vi "Write Configuration to File.vi"(8 "error in":errorcluster, 11 "?":T1={"Data Tree Ref"=refnum, "FP Ref"=refnum, "Column Data Type"=[], "Search Clones Up To"=0, "SortOptions"={"Col.pri"=0, "RevDir.pri"=FALSE, "Col.sec"=0, "RevDir.sec"=FALSE}, "Group/Flat (0:group)"=FALSE, "CollapsedNodes"=[], "Show/Hide Cols"=[], "Filtered Paths"=[], "View"=enum."Group By Library", "File Extension Filters"=[], "Filter Global VIs"=FALSE, "Shared"=refnum, "Active Filters"=refnum, "Refresh Rate (ms)"=2000}) -> (0 "error out":errorcluster)   [LabVIEW 2013, in "LVTM.lvlib"]
uses:
  LVTM.lvlib
  Controls_LVTM/LVTM_Config_Info.ctl
  Controls_LVTM/View.ctl
  Controls_LVTM/SharedDataDVR.ctl
  <vilib>/Utility/config.llb/Write Key (String).vi
  <vilib>/Utility/config.llb/Write Key (Boolean).vi
  <vilib>/Utility/config.llb/Write Key (I32).vi
  <vilib>/Utility/config.llb/Write Key (Path).vi
  <vilib>/Utility/config.llb/NI_LVConfig.lvlib
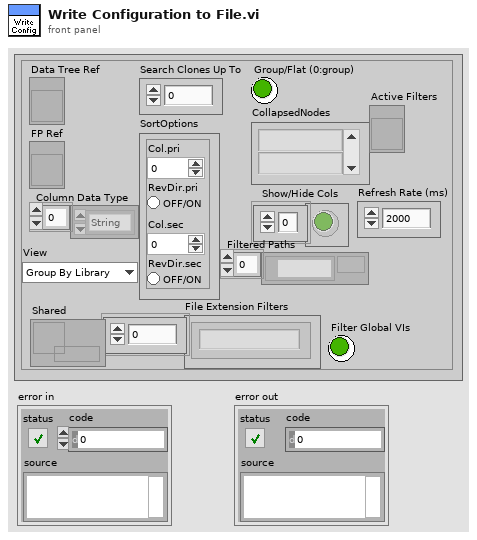
[diagram p1: front panel]
types:
  T1 = typedef "LVTM.lvlib/LVTM_Config_Info.ctl" = cluster{"Data Tree Ref":refnum<vi>, "FP Ref":refnum<vi>, "Column Data Type":enum16{"String", "Numeric"}[], "Search Clones Up To":i32, "SortOptions":cluster{"Col.pri":i32, "RevDir.pri":bool, "Col.sec":i32, "RevDir.sec":bool}, "Group/Flat (0:group)":bool, "CollapsedNodes":string[], "Show/Hide Cols":bool[], "Filtered Paths":path[], "View":T2, "File Extension Filters":string[], "Filter Global VIs":bool, "Shared":refnum<data-value>, "Active Filters":refnum<vi>, "Refresh Rate (ms)":i32}
  T2 = typedef "LVTM.lvlib/View.ctl" = enum16{"Group By Library", "Group By Folder", "Flat List"}
  T3 = typedef "NI_LVConfig.lvlib/Config Data RefNum.ctl" = refnum<k1>
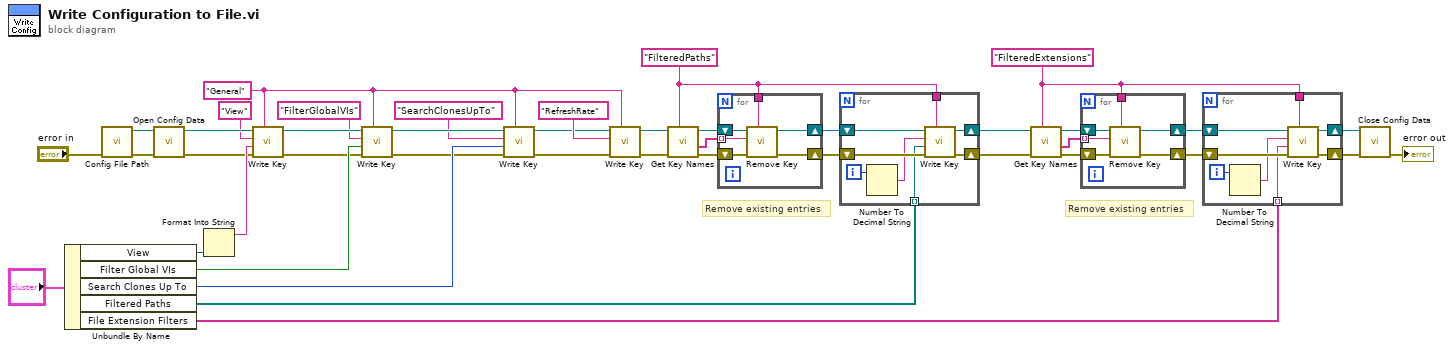
[diagram p0: block diagram]
diagram:
  w14 = "FilteredExtensions" ("section")
  w23 = "FilteredPaths" ("section")
  w4 = "General" ("section")
  # "Remove existing entries"
  # "Remove existing entries"
  n1 = Unbundle By Name("?") -> ("View"=w28:T2, "Filter Global VIs"=w39:bool, "Search Clones Up To"=w40:i32, "Filtered Paths"=w25:path[], "File Extension Filters"=w10:string[])
  n2 = call "Config File Path.vi"("error in"="error in") -> ("error out"=w27:errorcluster, "Config File Path"=w26:path)  [unwired: 9 in]
  n3 = call <vilib>:"Open Config Data.vi"("error in (no error)"=w27, "configuration file path"=w26) -> ("error out"=w29:errorcluster, "refnum"=w32:T3)  [unwired: 7 in, 1 out]
  n4 = Format Into String(w28) -> (resulting string=w30:string)  [unwired: 3 in, 1 out]
  n5 = call-poly <vilib>:"Write Key.vi"("section"=w4, "error in (no error)"=w29, "value"=w30, "key"="View", "refnum"=w32) -> ("error out"=w35:errorcluster, "refnum out"=w34:T3)  [unwired: 4 in, 1 out]
  n6 = call-poly <vilib>:"Write Key.vi"("section"=w4, "error in (no error)"=w35, "value"=w39, "key"="FilterGlobalVIs", "refnum"=w34) -> ("error out"=w38:errorcluster, "refnum out"=w37:T3)  [unwired: 4 in, 1 out]
  n7 = call-poly <vilib>:"Write Key.vi"("section"=w4, "error in (no error)"=w38, "value"=w40, "key"="SearchClonesUpTo", "refnum"=w37) -> ("error out"=w3:errorcluster, "refnum out"=w5:T3)  [unwired: 4 in, 1 out]
  n8 = call-poly <vilib>:"Write Key.vi"("section"=w4, "error in (no error)"=w3, "key"="RefreshRate", "refnum"=w5) -> ("error out"=w2:errorcluster, "refnum out"=w1:T3)  [unwired: 5 in, 1 out]
  n9 = call <vilib>:"Get Key Names.vi"("section"=w23, "error in (no error)"=w2, "refnum"=w1) -> ("error out"=w22:errorcluster, "key names"=w21:string[], "refnum out"=w24:T3)  [unwired: 5 in, 1 out]
  n10 = for {
    shift-right: [w46] -> w20
    shift-left: w24 -> [w47]
    shift-right: [w45] -> w19
    shift-left: w22 -> [w48]
    tunnel: w23 -> [w44]
    tunnel: w21 -> [w43] mode=indexing
    n11 = call <vilib>:"Remove Key.vi"("section"=w44, "error in (no error)"=w48, "key"=w43, "refnum"=w47) -> ("error out"=w45:errorcluster, "refnum out"=w46:T3)  [unwired: 5 in, 1 out]
  }
  n12 = for {
    shift-right: [w54] -> w12
    shift-left: w20 -> [w55]
    shift-right: [w53] -> w11
    shift-left: w19 -> [w56]
    tunnel: w25 -> [w52] mode=indexing
    tunnel: w23 -> [w49]
    i -> [w51]
    n13 = Number To Decimal String(number=w51) -> (decimal integer string=w50:string)  [unwired: 1 in]
    n14 = call-poly <vilib>:"Write Key.vi"("section"=w49, "error in (no error)"=w56, "value"=w52, "key"=w50, "refnum"=w55) -> ("error out"=w53:errorcluster, "refnum out"=w54:T3)  [unwired: 4 in, 1 out]
  }
  n15 = call <vilib>:"Get Key Names.vi"("section"=w14, "error in (no error)"=w11, "refnum"=w12) -> ("error out"=w15:errorcluster, "key names"=w16:string[], "refnum out"=w13:T3)  [unwired: 5 in, 1 out]
  n16 = for {
    shift-right: [w60] -> w17
    shift-left: w13 -> [w61]
    shift-right: [w59] -> w18
    shift-left: w15 -> [w62]
    tunnel: w14 -> [w58]
    tunnel: w16 -> [w57] mode=indexing
    n17 = call <vilib>:"Remove Key.vi"("section"=w58, "error in (no error)"=w62, "key"=w57, "refnum"=w61) -> ("error out"=w59:errorcluster, "refnum out"=w60:T3)  [unwired: 5 in, 1 out]
  }
  n18 = for {
    shift-right: [w68] -> w9
    shift-left: w17 -> [w69]
    shift-right: [w67] -> w8
    shift-left: w18 -> [w70]
    tunnel: w10 -> [w66] mode=indexing
    tunnel: w14 -> [w63]
    i -> [w65]
    n19 = Number To Decimal String(number=w65) -> (decimal integer string=w64:string)  [unwired: 1 in]
    n20 = call-poly <vilib>:"Write Key.vi"("section"=w63, "error in (no error)"=w70, "value"=w66, "key"=w64, "refnum"=w69) -> ("error out"=w67:errorcluster, "refnum out"=w68:T3)  [unwired: 4 in, 1 out]
  }
  n21 = call <vilib>:"Close Config Data.vi"("error in (no error)"=w8, "refnum"=w9) -> ("error out"=→"error out":errorcluster)  [unwired: 8 in, 1 out]
